vi "Measured Phase.vi"(10 "Total Phase":dbl, 11 "Measured Position":dbl[](array[numeric])) -> (3 "Measured Phase":dbl)   [LabVIEW 2021]
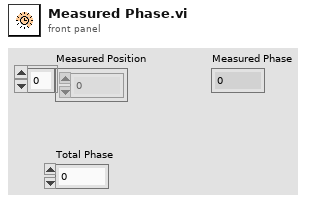
[diagram p1: front panel]
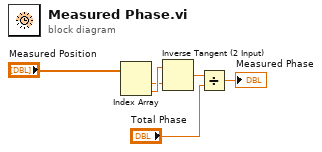
[diagram p0: block diagram]
diagram:
  n1 = Index Array(array="Measured Position") -> (element #1=w1:dbl, element #2=w2:dbl)  [unwired: 2 in]
  n2 = Inverse Tangent (2 Input)(1:w1, 2:w2) -> (0:w3:dbl)
  n3 = Divide(x=w3, y="Total Phase") -> (x/y=→"Measured Phase":dbl)
